vi "Test Asic Digital Offset modificar cluster.vi"(8 "Error IN":errorcluster, 11 "Config Test IN":T1={"Config HW"={"VISA Rigol DP832"="Rigol_DP832", "Config Rigol DP832"=[{"Channel"=0, "V Limit"=5.5, "I Limit"=0.5, "V Out"=5.0}, {"Channel"=1, "V Limit"=5.5, "I Limit"=0.8, "V Out"=5.0}, {"Channel"=2, "V Limit"=5.5, "I Limit"=0.2, "V Out"=0.0}], "CTA Test#"="CTA013 A", "FT_Handle"=0, "Espera acceso FT"=10}, "Config Test"=[{"Vasic"=3.3, "Test Register?"=TRUE, "Test ADC?"=TRUE, "Test ADC"={"Repeats ADC"=100, "Max Desviation"=0.1}, "Test Max PN Min NP?"=TRUE, "Limits Max PN Min NP"={"Max P inferior"=1.888, "Max P superior"=2.177000045776367, "Min N superior"=0.818, "Min N inferior"=0.73, "Max N superior"=1.475, "Max N inferior"=1.322, "Min P inferior "=1.321, "Min P superior"=1.474}, "Test Rate Scan?"=TRUE, "Vin Rate Scan"=[0, 1, 2, 3, 4, 5, 6, 7, 8, 9], "Limits Rate Scan"={"High"=[], "Low"=[]}, "Test Rate Scan Adders? 2"=FALSE, "Vin Rate Adders"=[], "Test offset analog?"=TRUE, "Test offset digital?"=FALSE, "Lim Offset Analog"={"Max Analog"=0.05, "Min Analog"=-0.05}, "Lim offset Dig"={"Max Dig"=0.05}}, {"Vasic"=3.2, "Test Register?"=TRUE, "Test ADC?"=TRUE, "Test ADC"={"Repeats ADC"=100, "Max Desviation"=0.1}, "Test Max PN Min NP?"=TRUE, "Limits Max PN Min NP"={"Max P inferior"=1.888, "Max P superior"=2.177000045776367, "Min N superior"=0.818, "Min N inferior"=0.73, "Max N superior"=1.475, "Max N inferior"=1.322, "Min P inferior "=1.321, "Min P superior"=1.474}, "Test Rate Scan?"=TRUE, "Vin Rate Scan"=[0, 3], "Limits Rate Scan"={"High"=[], "Low"=[]}, "Test Rate Scan Adders? 2"=FALSE, "Vin Rate Adders"=[], "Test offset analog?"=TRUE, "Test offset digital?"=FALSE, "Lim Offset Analog"={"Max Analog"=0.05, "Min Analog"=-0.05}, "Lim offset Dig"={"Max Dig"=0.05}}, {"Vasic"=3.1, "Test Register?"=TRUE, "Test ADC?"=TRUE, "Test ADC"={"Repeats ADC"=100, "Max Desviation"=0.1}, "Test Max PN Min NP?"=TRUE, "Limits Max PN Min NP"={"Max P inferior"=1.888, "Max P superior"=2.177000045776367, "Min N superior"=0.818, "Min N inferior"=0.73, "Max N superior"=1.475, "Max N inferior"=1.322, "Min P inferior "=1.321, "Min P superior"=1.474}, "Test Rate Scan?"=TRUE, "Vin Rate Scan"=[0, 3], "Limits Rate Scan"={"High"=[], "Low"=[]}, "Test Rate Scan Adders? 2"=FALSE, "Vin Rate Adders"=[], "Test offset analog?"=TRUE, "Test offset digital?"=FALSE, "Lim Offset Analog"={"Max Analog"=0.05, "Min Analog"=-0.05}, "Lim offset Dig"={"Max Dig"=0.05}}, {"Vasic"=3.0, "Test Register?"=TRUE, "Test ADC?"=TRUE, "Test ADC"={"Repeats ADC"=100, "Max Desviation"=0.1}, "Test Max PN Min NP?"=TRUE, "Limits Max PN Min NP"={"Max P inferior"=1.888, "Max P superior"=2.177000045776367, "Min N superior"=0.818, "Min N inferior"=0.73, "Max N superior"=1.475, "Max N inferior"=1.322, "Min P inferior "=1.321, "Min P superior"=1.474}, "Test Rate Scan?"=TRUE, "Vin Rate Scan"=[0, 3], "Limits Rate Scan"={"High"=[], "Low"=[]}, "Test Rate Scan Adders? 2"=FALSE, "Vin Rate Adders"=[], "Test offset analog?"=TRUE, "Test offset digital?"=FALSE, "Lim Offset Analog"={"Max Analog"=0.05, "Min Analog"=-0.05}, "Lim offset Dig"={"Max Dig"=0.05}}], "Result"=[], "Execucion Test"={"Vasic Actual"=0}, "Config VGA"={"Theoretical Voltage"=[], "Real Voltage"=[102.85, 207.14, 299.57, 404.85, 495.71, 606.85, 697.71, 801.14, 897.14, 998.85], "Pulse Width"=57344, "Frecuency Pulse"=1000000.0, "VGA Gain"=[9, 16, 24, 34, 43, 52, 61, 72, 81, 93]}, "Test Info"={"Asic"="", "Operator"="", "Time start"=timestamp(0 s since 1904-01-01), "Time stop"=timestamp(0 s since 1904-01-01)}} {"Config VGA"."Theoretical Voltage" format="%1.4f"; "Config VGA"."VGA Gain" format="%02x"; "Config VGA"."Frecuency Pulse" format="%0_2p"; "Config VGA"."Pulse Width" format="%04x"; "Config VGA"."Real Voltage" format="%1.5f"; "Config Test"."Lim offset Dig"."Max Dig" format="%.3g"; "Config Test"."Lim Offset Analog"."Min Analog" format="%.3g"; "Config Test"."Lim Offset Analog"."Max Analog" format="%.3g"; "Config Test"."Limits Rate Scan"."Low" format="%1.4f"; "Config Test"."Limits Rate Scan"."High" format="%1.3f"; "Config Test"."Limits Max PN Min NP"."Min P superior" format="%.3g"; "Config Test"."Limits Max PN Min NP"."Min P inferior" format="%.3g"; "Config Test"."Limits Max PN Min NP"."Max N inferior" format="%.3g"; "Config Test"."Limits Max PN Min NP"."Max N superior" format="%.3g"; "Config Test"."Limits Max PN Min NP"."Min N inferior" format="%.3g"; "Config Test"."Limits Max PN Min NP"."Min N superior" format="%.3g"; "Config Test"."Limits Max PN Min NP"."Max P superior" format="%.3g"; "Config Test"."Limits Max PN Min NP"."Max P inferior" format="%.3g"; "Config Test"."Vasic" min=2.8 max=3.8 step=0.01 format="%.2g"; "Config HW"."Config Rigol DP832"."Channel" items=["+30V Channel 1", "+30V Channel 2", "+5V Channel 3"]; "Config HW"."Config Rigol DP832"."V Limit" format="%.1g"; "Config HW"."Config Rigol DP832"."I Limit" format="%.1g"; "Config HW"."Config Rigol DP832"."V Out" format="%.1g"; "Result"."Test Registros"."Read W/R" format="%04x"; "Result"."Test Registros"."Pattern W/R" format="%04x"; "Result"."Test Registros"."Read Default" format="%04x"; "Result"."Test Registros"."Pattern Default" format="%04x"}) -> (0 "Error OUT":errorcluster, 3 "Config Test OUT":T1={"Config HW"={"VISA Rigol DP832"="Rigol_DP832", "Config Rigol DP832"=[{"Channel"=0, "V Limit"=5.5, "I Limit"=0.5, "V Out"=5.0}, {"Channel"=1, "V Limit"=5.5, "I Limit"=0.8, "V Out"=5.0}, {"Channel"=2, "V Limit"=5.5, "I Limit"=0.2, "V Out"=0.0}], "CTA Test#"="CTA013 A", "FT_Handle"=0, "Espera acceso FT"=10}, "Config Test"=[{"Vasic"=3.3, "Test Register?"=TRUE, "Test ADC?"=TRUE, "Test ADC"={"Repeats ADC"=100, "Max Desviation"=0.1}, "Test Max PN Min NP?"=TRUE, "Limits Max PN Min NP"={"Max P inferior"=1.888, "Max P superior"=2.177000045776367, "Min N superior"=0.818, "Min N inferior"=0.73, "Max N superior"=1.475, "Max N inferior"=1.322, "Min P inferior "=1.321, "Min P superior"=1.474}, "Test Rate Scan?"=TRUE, "Vin Rate Scan"=[0, 1, 2, 3, 4, 5, 6, 7, 8, 9], "Limits Rate Scan"={"High"=[], "Low"=[]}, "Test Rate Scan Adders? 2"=FALSE, "Vin Rate Adders"=[], "Test offset analog?"=TRUE, "Test offset digital?"=FALSE, "Lim Offset Analog"={"Max Analog"=0.05, "Min Analog"=-0.05}, "Lim offset Dig"={"Max Dig"=0.05}}, {"Vasic"=3.2, "Test Register?"=TRUE, "Test ADC?"=TRUE, "Test ADC"={"Repeats ADC"=100, "Max Desviation"=0.1}, "Test Max PN Min NP?"=TRUE, "Limits Max PN Min NP"={"Max P inferior"=1.888, "Max P superior"=2.177000045776367, "Min N superior"=0.818, "Min N inferior"=0.73, "Max N superior"=1.475, "Max N inferior"=1.322, "Min P inferior "=1.321, "Min P superior"=1.474}, "Test Rate Scan?"=TRUE, "Vin Rate Scan"=[0, 3], "Limits Rate Scan"={"High"=[], "Low"=[]}, "Test Rate Scan Adders? 2"=FALSE, "Vin Rate Adders"=[], "Test offset analog?"=TRUE, "Test offset digital?"=FALSE, "Lim Offset Analog"={"Max Analog"=0.05, "Min Analog"=-0.05}, "Lim offset Dig"={"Max Dig"=0.05}}, {"Vasic"=3.1, "Test Register?"=TRUE, "Test ADC?"=TRUE, "Test ADC"={"Repeats ADC"=100, "Max Desviation"=0.1}, "Test Max PN Min NP?"=TRUE, "Limits Max PN Min NP"={"Max P inferior"=1.888, "Max P superior"=2.177000045776367, "Min N superior"=0.818, "Min N inferior"=0.73, "Max N superior"=1.475, "Max N inferior"=1.322, "Min P inferior "=1.321, "Min P superior"=1.474}, "Test Rate Scan?"=TRUE, "Vin Rate Scan"=[0, 3], "Limits Rate Scan"={"High"=[], "Low"=[]}, "Test Rate Scan Adders? 2"=FALSE, "Vin Rate Adders"=[], "Test offset analog?"=TRUE, "Test offset digital?"=FALSE, "Lim Offset Analog"={"Max Analog"=0.05, "Min Analog"=-0.05}, "Lim offset Dig"={"Max Dig"=0.05}}, {"Vasic"=3.0, "Test Register?"=TRUE, "Test ADC?"=TRUE, "Test ADC"={"Repeats ADC"=100, "Max Desviation"=0.1}, "Test Max PN Min NP?"=TRUE, "Limits Max PN Min NP"={"Max P inferior"=1.888, "Max P superior"=2.177000045776367, "Min N superior"=0.818, "Min N inferior"=0.73, "Max N superior"=1.475, "Max N inferior"=1.322, "Min P inferior "=1.321, "Min P superior"=1.474}, "Test Rate Scan?"=TRUE, "Vin Rate Scan"=[0, 3], "Limits Rate Scan"={"High"=[], "Low"=[]}, "Test Rate Scan Adders? 2"=FALSE, "Vin Rate Adders"=[], "Test offset analog?"=TRUE, "Test offset digital?"=FALSE, "Lim Offset Analog"={"Max Analog"=0.05, "Min Analog"=-0.05}, "Lim offset Dig"={"Max Dig"=0.05}}], "Result"=[], "Execucion Test"={"Vasic Actual"=0}, "Config VGA"={"Theoretical Voltage"=[], "Real Voltage"=[102.85, 207.14, 299.57, 404.85, 495.71, 606.85, 697.71, 801.14, 897.14, 998.85], "Pulse Width"=57344, "Frecuency Pulse"=1000000.0, "VGA Gain"=[9, 16, 24, 34, 43, 52, 61, 72, 81, 93]}, "Test Info"={"Asic"="", "Operator"="", "Time start"=timestamp(0 s since 1904-01-01), "Time stop"=timestamp(0 s since 1904-01-01)}} {"Config VGA"."Theoretical Voltage" format="%1.4f"; "Config VGA"."VGA Gain" format="%02x"; "Config VGA"."Frecuency Pulse" format="%0_2p"; "Config VGA"."Pulse Width" format="%04x"; "Config VGA"."Real Voltage" format="%1.5f"; "Config Test"."Lim offset Dig"."Max Dig" format="%.3g"; "Config Test"."Lim Offset Analog"."Min Analog" format="%.3g"; "Config Test"."Lim Offset Analog"."Max Analog" format="%.3g"; "Config Test"."Limits Rate Scan"."Low" format="%1.4f"; "Config Test"."Limits Rate Scan"."High" format="%1.3f"; "Config Test"."Limits Max PN Min NP"."Min P superior" format="%.3g"; "Config Test"."Limits Max PN Min NP"."Min P inferior" format="%.3g"; "Config Test"."Limits Max PN Min NP"."Max N inferior" format="%.3g"; "Config Test"."Limits Max PN Min NP"."Max N superior" format="%.3g"; "Config Test"."Limits Max PN Min NP"."Min N inferior" format="%.3g"; "Config Test"."Limits Max PN Min NP"."Min N superior" format="%.3g"; "Config Test"."Limits Max PN Min NP"."Max P superior" format="%.3g"; "Config Test"."Limits Max PN Min NP"."Max P inferior" format="%.3g"; "Config Test"."Vasic" min=2.8 max=3.8 step=0.01 format="%.2g"; "Config HW"."Config Rigol DP832"."Channel" items=["+30V Channel 1", "+30V Channel 2", "+5V Channel 3"]; "Config HW"."Config Rigol DP832"."V Limit" format="%.1g"; "Config HW"."Config Rigol DP832"."I Limit" format="%.1g"; "Config HW"."Config Rigol DP832"."V Out" format="%.1g"; "Result"."Test Registros"."Read W/R" format="%04x"; "Result"."Test Registros"."Pattern W/R" format="%04x"; "Result"."Test Registros"."Read Default" format="%04x"; "Result"."Test Registros"."Pattern Default" format="%04x"})   [LabVIEW 2009]
uses:
  Test.ctl
  TEST.TEST CONFIG HW.ctl
  Rigol DP832/DP832_Control Channels.ctl
  TEST.TEST CONFIG TEST MATRIZ.ctl
  TEST.TEST CONFIG TEST.ctl
  TEST.TEST RESULT.ctl
  test_result fvasic.ctl
  TEST.TEST EXECUTION TEST.ctl
  TEST.TEST CONFIG VGA.ctl
  TEST.TEST TEST INFO.ctl
panel:
  out "REF":cluster{"Sumador":u8, "Canal":u8}
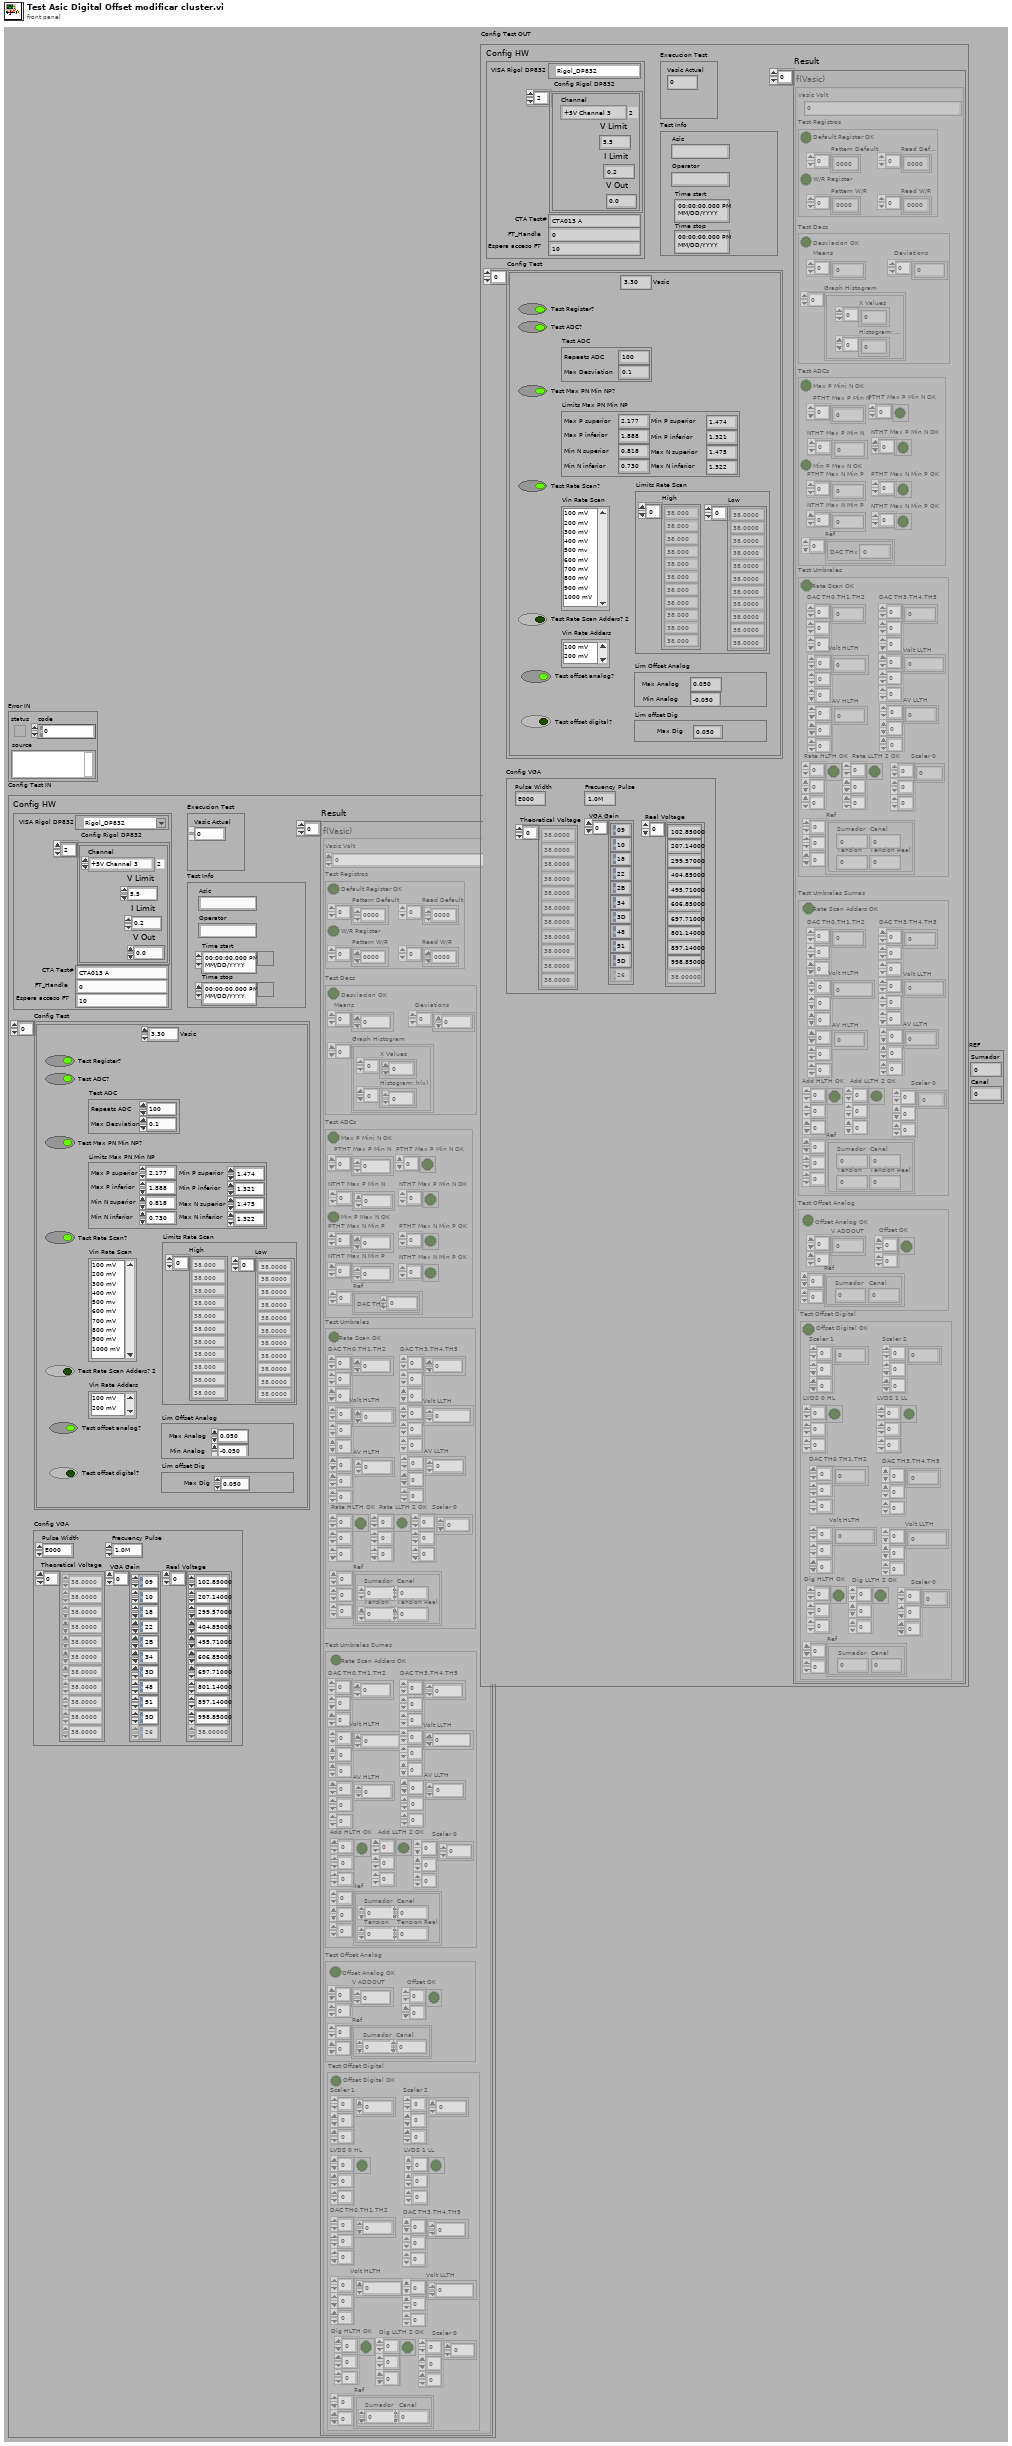
[diagram p1: front panel]
types:
  T1 = typedef "Test.ctl" = cluster{"Config HW":T2, "Config Test":T4, "Result":T6, "Execucion Test":T8, "Config VGA":T9, "Test Info":T10}
  T2 = typedef "TEST.TEST CONFIG HW.ctl" = cluster{"VISA Rigol DP832":refnum<visa-resource-name>, "Config Rigol DP832":cluster{"Channel":T3, "V Limit":dbl, "I Limit":dbl, "V Out":dbl}[], "CTA Test#":string, "FT_Handle":u32, "Espera acceso FT":u32}
  T3 = typedef "DP832_Control Channels.ctl" = i32
  T4 = typedef "TEST.TEST CONFIG TEST MATRIZ.ctl" = T5[]
  T5 = typedef "TEST.TEST CONFIG TEST.ctl" = cluster{"Vasic":dbl, "Test Register?":bool, "Test ADC?":bool, "Test ADC":cluster{"Repeats ADC":i32, "Max Desviation":dbl}, "Test Max PN Min NP?":bool, "Limits Max PN Min NP":cluster{"Max P inferior":dbl, "Max P superior":dbl, "Min N superior":dbl, "Min N inferior":dbl, "Max N superior":dbl, "Max N inferior":dbl, "Min P inferior ":dbl, "Min P superior":dbl}, "Test Rate Scan?":bool, "Vin Rate Scan":i32[], "Limits Rate Scan":cluster{"High":dbl[], "Low":dbl[]}, "Test Rate Scan Adders? 2":bool, "Vin Rate Adders":i32[], "Test offset analog?":bool, "Test offset digital?":bool, "Lim Offset Analog":cluster{"Max Analog":dbl, "Min Analog":dbl}, "Lim offset Dig":cluster{"Max Dig":dbl}}
  T6 = typedef "TEST.TEST RESULT.ctl" = T7[]
  T7 = typedef "test_result fvasic.ctl" = cluster{"Vasic Volt":i32, "Test Registros":cluster{"Default Register OK":bool, "Pattern Default":u16[], "Read Default":u16[], "W/R Register":bool, "Pattern W/R":u16[], "Read W/R":u16[]}, "Test Dacs":cluster{"Desviacion OK":bool, "Means":dbl[], "Deviations":dbl[], "Graph Histogram":cluster{"X Values":dbl[], "Histogram: h(x)":i32[]}[]}, "Test ADCs":cluster{"Max P Mini N OK":bool, "PTHT Max P Min N":dbl[], "PTHT Max P Min N OK":bool[], "NTHT Max P Min N":dbl[], "NTHT Max P Min N OK":bool[], "Min P Max N OK":bool, "PTHT Max N Min P":dbl[], "PTHT Max N Min P OK":bool[], "NTHT Max N Min P":dbl[], "NTHT Max N Min P OK":bool[], "Ref":cluster{"DAC THx":u8}[]}, "Test Umbrales":cluster{"Rate Scan OK":bool, "DAC TH0,TH1,TH2":u16[][][], "Volt HLTH":dbl[][][], "AV HLTH":dbl[][][], "Rate HLTH OK":bool[][][], "DAC TH3,TH4,TH5":u16[][][], "Volt LLTH":dbl[][][], "AV LLTH":dbl[][][], "Rate LLTH 2 OK":bool[][][], "Scaler 0":u16[][][], "Ref":cluster{"Sumador":u8, "Canal":u8, "Tension":u8, "Tension Real":dbl}[][][]}, "Test Umbrales Sumas":cluster{"Rate Scan Adders OK":bool, "DAC TH0,TH1,TH2":u16[][][], "Volt HLTH":dbl[][][], "AV HLTH":dbl[][][], "Add HLTH OK":bool[][][], "DAC TH3,TH4,TH5":u16[][][], "Volt LLTH":dbl[][][], "AV LLTH":dbl[][][], "Add LLTH 2 OK":bool[][][], "Scaler 0":u16[][][], "Ref":cluster{"Sumador":u8, "Canal":u8, "Tension":u8, "Tension Real":dbl}[][][]}, "Test Offset Analog":cluster{"Offset Analog OK":bool, "V ADDOUT":dbl[][], "Offset OK":bool[][], "Ref":cluster{"Sumador":u8, "Canal":u8}[][]}, "Test Offset Digital":cluster{"Offset Digital OK":bool, "Scaler 1":u16[][][], "LVDS 0 HL":bool[][][], "DAC TH0,TH1,TH2":u16[][][], "Volt HLTH":dbl[][][], "Dig HLTH OK":bool[][][], "Scaler 2":u16[][][], "LVDS 1 LL":bool[][][], "DAC TH3,TH4,TH5":u16[][][], "Volt LLTH":dbl[][][], "Dig LLTH 2 OK":bool[][][], "Scaler 0":u16[][][], "Ref":cluster{"Sumador":u8, "Canal":u8}[][]}}
  T8 = typedef "TEST.TEST EXECUTION TEST.ctl" = cluster{"Vasic Actual":i32}
  T9 = typedef "TEST.TEST CONFIG VGA.ctl" = cluster{"Theoretical Voltage":dbl[], "Real Voltage":dbl[], "Pulse Width":u16, "Frecuency Pulse":dbl, "VGA Gain":u8[]}
  T10 = typedef "TEST.TEST TEST INFO.ctl" = cluster{"Asic":string, "Operator":string, "Time start":timestamp, "Time stop":timestamp}
  T11 = cluster{"SCALER 0":u16[], "SCALER 1":u16[], "LVDS 1 HL":bool[], "THX":u16[], "VHLTH":dbl[], "SCALER 2":u16[], "LVDS 2 LL":bool[], "THX+3":u16[], "VLLTH":dbl[]}
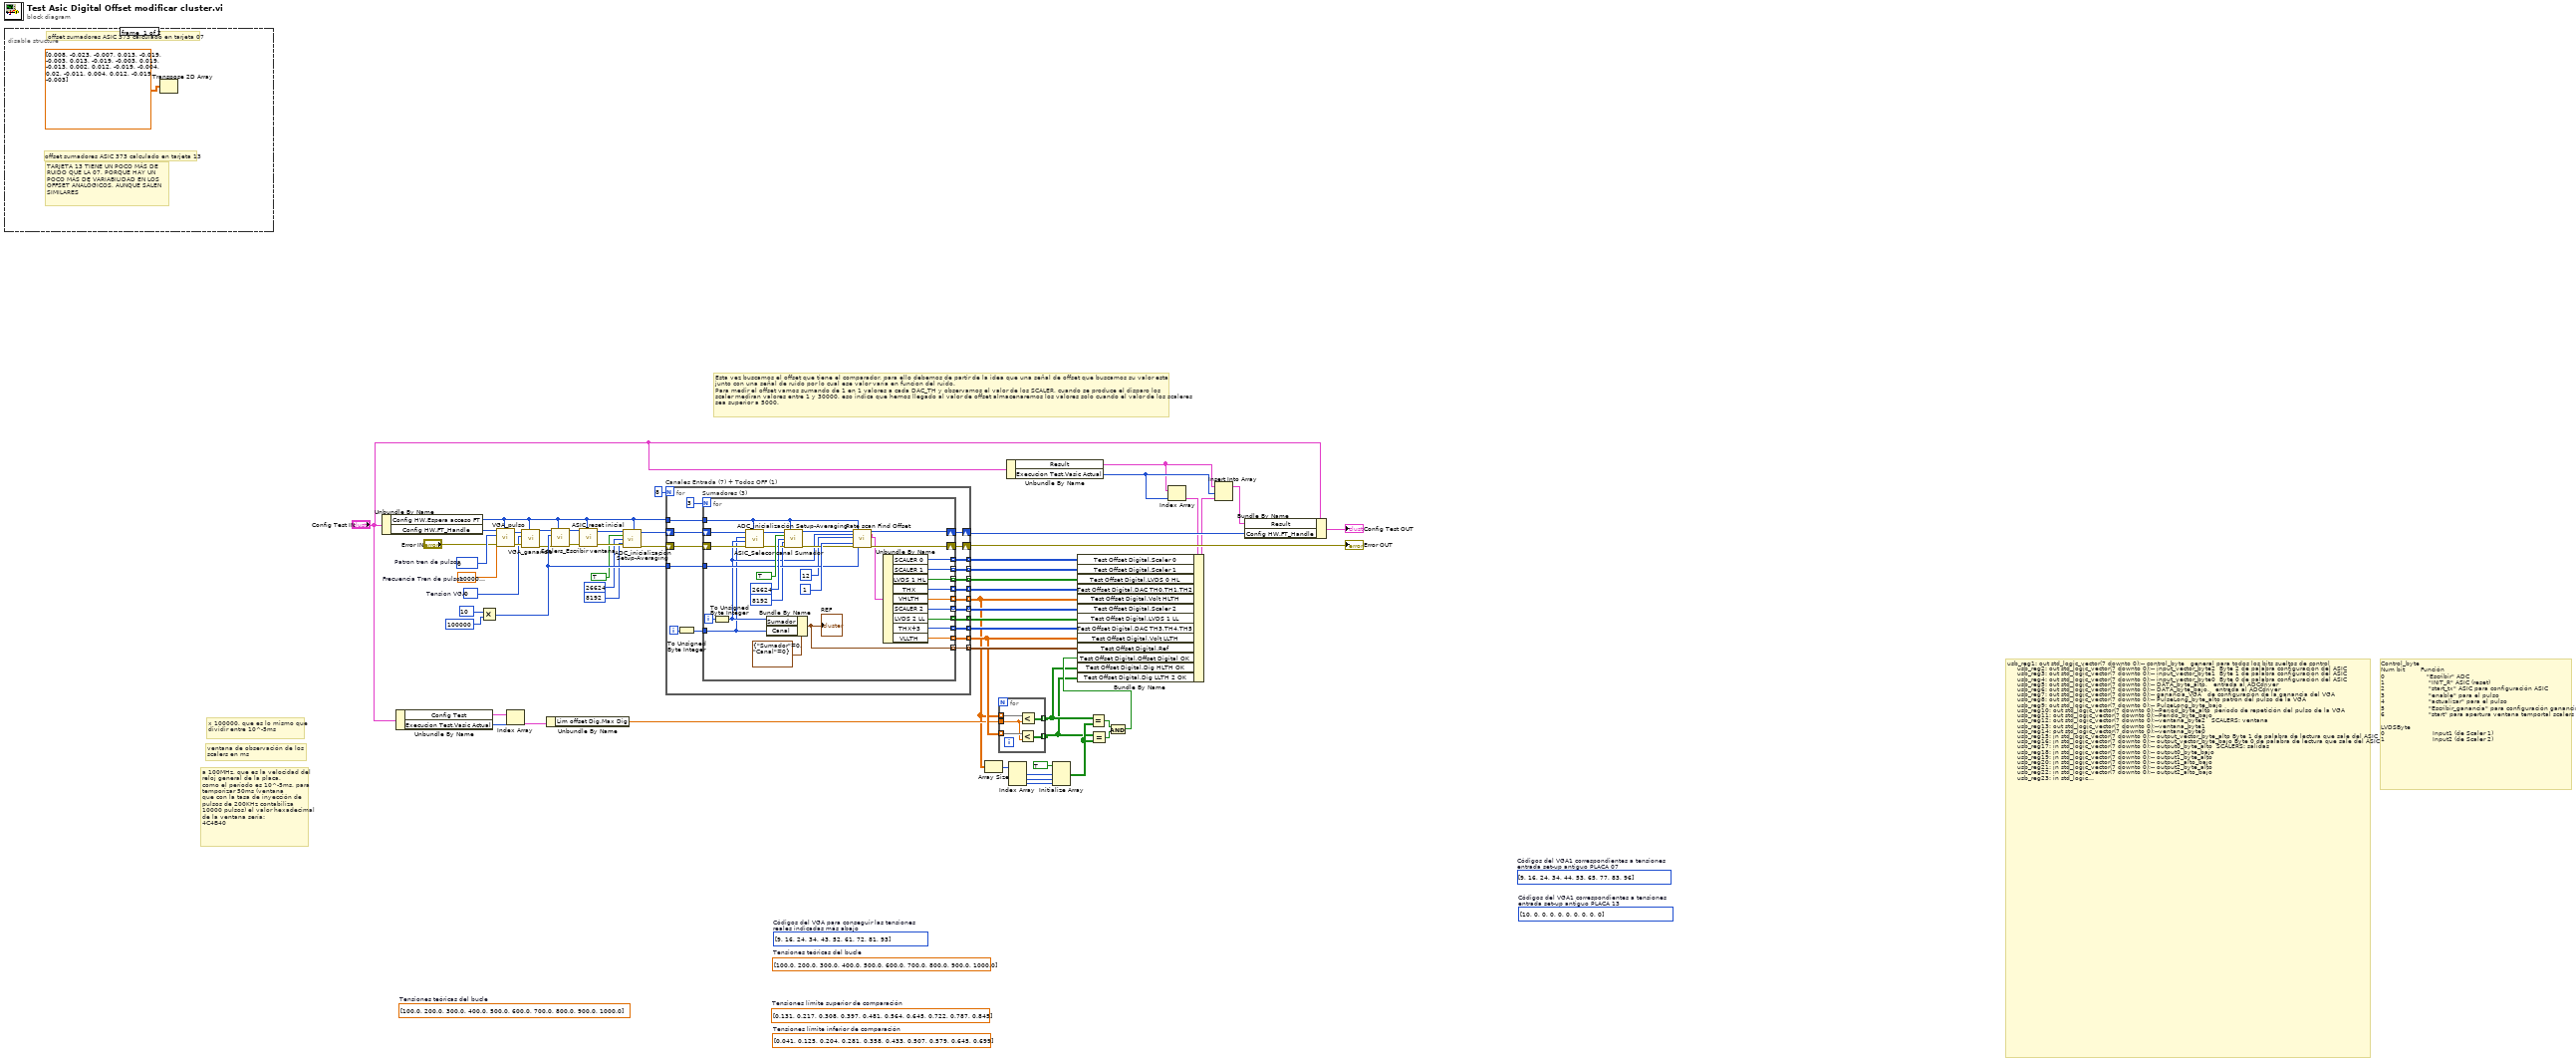
[diagram p0: block diagram]
diagram:
  w37 = u8 0  # Tension VGA
  (unwired) dbl[] [100.0, 200.0, 300.0, 400.0, 500.0, 600.0, 700.0, 800.0, 900.0, 1000.0]  # Tensiones teóricas del bucle
  w51 = 1000000.0  # Frecuencia Tren de pulsos
  w52 = u16 0  # Patron tren de pulsos
  (unwired) u8[] [10, 0, 0, 0, 0, 0, 0, 0, 0, 0]  # Códigos del VGA1 correspondientes a tensiones entrada set-up antiguo PLACA 13
  (unwired) u8[] [9, 16, 24, 34, 44, 53, 65, 77, 83, 96]  # Códigos del VGA1 correspondientes a tensiones entrada set-up antiguo PLACA 07
  (unwired) u8[] [9, 16, 24, 34, 43, 52, 61, 72, 81, 93]  # Códigos del VGA para conseguir las tensiones reales indicadas más abajo
  (unwired) dbl[] [0.041, 0.125, 0.204, 0.281, 0.358, 0.433, 0.507, 0.579, 0.645, 0.699]  # Tensiones límite inferior de comparación
  (unwired) dbl[] [0.131, 0.217, 0.308, 0.397, 0.481, 0.564, 0.645, 0.722, 0.787, 0.845]  # Tensiones límite superior de comparación
  (unwired) dbl[] [100.0, 200.0, 300.0, 400.0, 500.0, 600.0, 700.0, 800.0, 900.0, 1000.0]  # Tensiones teóricas del bucle
  # "Esta vez buscamos el offset que tiene el comparador, para ello debemos de partir de la idea que una señal de offset que buscamos su valor esta\njunto con una señal de ruido por lo cual ese valor varia en funcion del ruido.\nPara medir el offset vamos sumando de 1 en 1 valores a cada DAC_TH y observamos el valor de los SCALER, cuando se produce el disparo los\nscaler mediran valores entre 1 y 30000, eso indica que hemos llegado al valor de offset almacenaremos los valores solo cuando el valor de los scaleres\nsea superior a 5000."
  # "Control_byte\nNum bit        Función\n0                     \"Escribir\" ADC\n1                      \"INIT_R\" ASIC (reset)\n2                      \"start_tx\" ASIC para configuración ASIC\n3                      \"enable\" para el pulso\n4                      \"actualizar\" para el pulso\n5                      \"Escribir_ganancia\" para configuración ganancia\n6                      \"start\" para apertura ventana temportal scalers\n\nLVDSByte\n0                        Input1 (de Scaler 1)\n1                        Input2 (de Scaler 2)"
  # "usb_reg1: out std_logic_vector(7 downto 0);-- control_byte\t\t\tgeneral para todos los bits sueltos de control\n\t\t\t  usb_reg2: out std_logic_vector(7 downto 0);-- input_vector_byte2 \tByte 2 de palabra configuración del ASIC\n\t\t\t  usb_reg3: out std_logic_vector(7 downto 0);-- input_vector_byte1 \tByte 1 de palabra configuración del ASIC\n\t\t\t  usb_reg4: out std_logic_vector(7 downto 0);-- input_vector_byte0 \tByte 0 de palabra configuración del ASIC\n\t\t\t  usb_reg5: out std_logic_vector(7 downto 0);-- DATA_byte_alto, \t\tentrada al ADCdriver\n\t\t\t  usb_reg6: out std_logic_vector(7 downto 0);-- DATA_byte_bajo, \t\tentrada al ADCdriver\n\t\t\t  usb_reg7: out std_logic_vector(7 downto 0);-- ganancia_VGA\t\t\tde configuración de la ganancia del VGA\n\t\t\t  usb_reg8: out std_logic_vector(7 downto 0);-- PulseLong_byte_alto\tpatrón del pulso de la VGA\n\t\t\t  usb_reg9: out std_logic_vector(7 downto 0);-- PulseLong_byte_bajo\n\t\t\t  usb_reg10: out std_logic_vector(7 downto 0);--Period_byte_alto\t\tperíodo de repetición del pulso de la VGA\n\t\t\t  usb_reg11: out std_logic_vector(7 downto 0);--Perido_byte_bajo\n\t\t\t  usb_reg12: out std_logic_vector(7 downto 0);--ventana_byte2\t\t\tSCALERS: ventana\n\t\t\t  usb_reg13: out std_logic_vector(7 downto 0);--ventana_byte1\t\n\t\t\t  usb_reg14: out std_logic_vector(7 downto 0);--ventana_byte0\n\t\t\t  usb_reg15: in std_logic_vector(7 downto 0);-- output_vector_byte_alto\tByte 1 de palabra de lectura que sale del ASIC\n\t\t\t  usb_reg16: in std_logic_vector(7 downto 0);-- output_vector_byte_bajo\tByte 0 de palabra de lectura que sale del ASIC\n\t\t\t  usb_reg17: in std_logic_vector(7 downto 0);-- output0_byte_alto\t\tSCALERS: salidas\n\t\t\t  usb_reg18: in std_logic_vector(7 downto 0);-- output0_byte_bajo\n\t\t\t  usb_reg19: in std_logic_vector(7 downto 0);-- output1_byte_alto\n\t\t\t  usb_reg20: in std_logic_vector(7 downto 0);-- output1_alto_bajo \n\t\t\t  usb_reg21: in std_logic_vector(7 downto 0);-- output2_byte_alto \n\t\t\t  usb_reg22: in std_logic_vector(7 downto 0);-- output2_alto_bajo \n\t\t\t  usb_reg23: in std_logic_vector(7 downto 0);-- para el canal_0 del ADCdriver\n\t\t\t  usb_reg24: in std_logic_vector(7 downto 0);\n\t\t\t  usb_reg25: in std_logic_vector(7 downto 0);-- para el canal_1 del ADCdriver\n\t\t\t  usb_reg26: in std_logic_vector(7 downto 0);\n\t\t\t  usb_reg27: in std_logic_vector(7 downto 0);-- para el canal_2 del ADCdriver\n\t\t\t  usb_reg28: in std_logic_vector(7 downto 0);\n\t\t\t  usb_reg29: in std_logic_vector(7 downto 0);-- para el canal_3 del ADCdriver\n\t\t\t  usb_reg30: in std_logic_vector(7 downto 0);\n\t\t\t  usb_reg31: in std_logic_vector(7 downto 0);-- para el canal_4 del ADCdriver\n\t\t\t  usb_reg32: in std_logic_vector(7 downto 0);\n\t\t\t  usb_reg33: in std_logic_vector(7 downto 0);-- para el canal_5 del ADCdriver\n\t\t\t  usb_reg34: in std_logic_vector(7 downto 0);\n\t\t\t  usb_reg35: in std_logic_vector(7 downto 0);-- para el canal_6 del ADCdriver\n\t\t\t  usb_reg36: in std_logic_vector(7 downto 0);\n\t\t\t  usb_reg37: in std_logic_vector(7 downto 0);-- para el canal_7 del ADCdriver\n\t\t\t  usb_reg38: in std_logic_vector(7 downto 0);\n\t\t\t  usb_reg39: in std_logic_vector(7 downto 0);-- para el canal_8 del ADCdriver\n\t\t\t  usb_reg40: in std_logic_vector(7 downto 0);\n\t\t\t  usb_reg41: in std_logic_vector(7 downto 0);-- para el canal_9 del ADCdriver\n\t\t\t  usb_reg42: in std_logic_vector(7 downto 0);\n\t\t\t  usb_reg43: in std_logic_vector(7 downto 0);-- para el canal_10 del ADCdriver\n\t\t\t  usb_reg44: in std_logic_vector(7 downto 0)--;  \n\n     usb_reg55 => LVDSByte"
  # "x 100000, que es lo mismo que dividir entre 10^-5ms"
  # "ventana de observación de los scalers en ms"
  # "a 100MHz, que es la velocidad del reloj general de la placa,\ncomo el período es 10^-5ms, para temporizar 50ms (ventana \nque con la tasa de inyección de pulsos de 200KHz contabiliza \n10000 pulsos) el valor hexadecimal de la ventana sería:\n4C4B40"
  n1 = disable-structure shown="Enabled" {
    frame #0 {
      # "TARJETA 13 TIENE UN POCO MÁS DE \nRUIDO QUE LA 07, PORQUE HAY UN\nPOCO MÁS DE VARIABILIDAD EN LOS \nOFFSET ANALÓGICOS, AUNQUE SALEN\nSIMILARES"
      # "offset sumadores ASIC 373 calculado en tarjeta 13"
      # "offset sumadores ASIC 373 calculado en tarjeta 07"
      n2 = Transpose 2D Array(2D array=dbl[][] [[0.008, -0.023, -0.007], [0.013, -0.019, -0.003], [0.013, -0.019, -0.003], [0.019, -0.013, 0.002], [0.012, -0.019, -0.004], [0.02, -0.011, 0.004], [0.012, -0.019, -0.003]]) -> ()  [unwired: 1 out]
    }
    frame #1 {
    }
  }
  n3 = Unbundle By Name("Config Test IN") -> ("Config HW.Espera acceso FT"=w38:u32, "Config HW.FT_Handle"=w50:u32)
  n4 = Unbundle By Name("Config Test IN") -> ("Config Test"=w16:T4, "Execucion Test.Vasic Actual"=w17:i32)
  n5 = Multiply(x=u32 10 ("Ventana"), y=u32 100000 ("Ventana")) -> (x*y=w53:u32)
  n6 = call "VGA_pulso.vi"("Espera acceso USB"=w38, "error in"="Error IN", "Frecuencia pulso (0.2 a 1 Mhz)"=w51, "Patrón (E000)"=w52, "ftHandle_in"=w50) -> ("error out"=w42:errorcluster, "ftHandle_out"=w39:u32)  [unwired: 5 in]
  n7 = Index Array(array=w16, index=w17) -> (element=w15:T5)
  n8 = call "VGA_ganancia.vi"("Espera acceso USB"=w38, "error in 2"=w42, "Ganancia"=w37, "ftHandle_in 2"=w39) -> ("error out 2"=w41:errorcluster, "ftHandle_out 2"=w40:u32)  [unwired: 6 in]
  n9 = Unbundle By Name(w15) -> ("Lim offset Dig.Max Dig"=w13:dbl)
  n10 = call "Scalers_Escribir ventana.vi"("Espera acceso USB"=w38, "error in"=w41, "Ventana"=w53, "ftHandle_in"=w40) -> ("error out"=w54:errorcluster, "ftHandle_out"=w55:u32)  [unwired: 6 in]
  n11 = call "ASIC_reset inicial.vi"("Espera acceso USB"=w38, "error in"=w54, "ftHandle_in"=w55) -> ("error out"=w47:errorcluster, "ftHandle_out"=w48:u32)  [unwired: 7 in]
  n12 = call "ADC_inicialización Setup-Averaging.vi"("ftHandle_in 2"=w48, "Espera acceso USB"=w38, "Reset (T=reset)"=TRUE, "Registro Setup (0x6800)"=u16 26624, "Registro Averaging (0x3200)"=u16 8192 ("Registro Setup (0x6800)"), "error in 2"=w47) -> ("ftHandle_out"=w32:u32, "error out"=w31:errorcluster)  [unwired: 8 in]
  n13 = for "Canales Entrada (7) + Todos OFF (1)" {
    N: 8 -> [_]
    tunnel: w38 -> [w73]
    tunnel: w53 -> [w74]
    shift-right: [w70] -> w45
    shift-left: w32 -> [w77]
    shift-right: [w69] -> w46
    shift-left: w31 -> [w76]
    tunnel: [w68] -> w27 mode=indexing
    tunnel: [w67] -> w26 mode=indexing
    tunnel: [w66] -> w25 mode=indexing
    tunnel: [w65] -> w24 mode=indexing
    tunnel: [w64] -> w7 mode=indexing
    tunnel: [w63] -> w23 mode=indexing
    tunnel: [w62] -> w22 mode=indexing
    tunnel: [w61] -> w21 mode=indexing
    tunnel: [w60] -> w14 mode=indexing
    tunnel: [w59] -> w20 mode=indexing
    i -> [w75]
    n14 = To Unsigned Byte Integer(number=w75) -> (unsigned 8bit integer=w71:u8)
    n15 = for "Sumadores (3)" {
      N: 3 -> [_]
      tunnel: w71 -> [w79]
      tunnel: w74 -> [w101]
      tunnel: w73 -> [w96]
      shift-right: [w93] -> w69
      shift-left: w76 -> [w100]
      shift-right: [w94] -> w70
      shift-left: w77 -> [w99]
      tunnel: [w90] -> w68 mode=indexing
      tunnel: [w89] -> w67 mode=indexing
      tunnel: [w88] -> w66 mode=indexing
      tunnel: [w87] -> w65 mode=indexing
      tunnel: [w86] -> w64 mode=indexing
      tunnel: [w85] -> w63 mode=indexing
      tunnel: [w84] -> w62 mode=indexing
      tunnel: [w83] -> w61 mode=indexing
      tunnel: [w82] -> w60 mode=indexing
      tunnel: [w78] -> w59 mode=indexing
      i -> [w106]
      n16 = To Unsigned Byte Integer(number=w106) -> (unsigned 8bit integer=w80:u8)
      n17 = call "ASIC_Selecor canal Sumador.vi"("Espera acceso USB"=w96, "error in"=w100, "Sumador"=w80, "Canal"=w79, "ftHandle_in"=w99) -> ("error out"=w98:errorcluster, "ftHandle_out"=w97:u32)  [unwired: 4 in, 1 out]
      n18 = Bundle By Name(cluster=cluster{"Sumador":u8, "Canal":u8} {"Sumador"=0, "Canal"=0}, "Sumador"=w80, "Canal"=w79) -> (w78:cluster{"Sumador":u8, "Canal":u8})
      "REF" <- w78
      n19 = call "ADC_inicialización Setup-Averaging.vi"("ftHandle_in 2"=w97, "Espera acceso USB"=w96, "Reset (T=reset)"=TRUE, "Registro Setup (0x6800)"=u16 26624, "Registro Averaging (0x3200)"=u16 8192 ("Registro Setup (0x6800)"), "error in 2"=w98) -> ("ftHandle_out"=w103:u32, "error out"=w102:errorcluster)  [unwired: 8 in]
      n20 = call "Rate scan Find Offset.vi"("FtHander IN"=w103, "Sumador"=w80, "Max Recorido Dac"=12, "Valor buscado scalers (5000)"=u16 1 ("Valor buscado scalers"), "Error IN"=w102, "Espera acceso USB"=w96, "T Ventana"=w101) -> ("FtHander OUT"=w94:u32, "Todos los valores"=w91:T11, "Error OUT"=w93:errorcluster)  [unwired: 9 in, 1 out]
      n21 = Unbundle By Name(w91) -> ("SCALER 0"=w90:u16[], "SCALER 1"=w89:u16[], "LVDS 1 HL"=w88:bool[], "THX"=w87:u16[], "VHLTH"=w86:dbl[], "SCALER 2"=w85:u16[], "LVDS 2 LL"=w84:bool[], "THX+3"=w83:u16[], "VLLTH"=w82:dbl[])
    }
  }
  "Error OUT" <- w46
  n22 = Array Size(array=w7) -> (size(s)=w12:i32[])
  n23 = for {
    tunnel: w7 -> [w112] mode=indexing
    tunnel: w14 -> [w111] mode=indexing
    tunnel: w13 -> [w110]
    tunnel: [w109] -> w2 mode=indexing
    tunnel: [w108] -> w1 mode=indexing
    n24 = Less?(x=w111, y=w110) -> (x < y?=w108:bool[][])
    n25 = Less?(x=w112, y=w110) -> (x < y?=w109:bool[][])
  }
  n26 = Unbundle By Name("Config Test IN") -> ("Result"=w30:T6, "Execucion Test.Vasic Actual"=w43:i32)
  n27 = Index Array(array=w12) -> (element #1=w11:i32, element #2=w10:i32, element #3=w9:i32)  [unwired: 3 in]
  n28 = Initialize Array(TRUE, w11, w10, w9) -> (w4:bool[][][])
  n29 = Equal?(x=w2, y=w4) -> (x = y?=w6:bool)
  n30 = Equal?(x=w1, y=w4) -> (x = y?=w5:bool)
  n31 = And(x=w6, y=w5) -> (x .and. y?=w3:bool)
  n32 = Index Array(array=w30, index=w43) -> (element=w28:T7)
  n33 = Bundle By Name(cluster=w28, "Test Offset Digital.Scaler 0"=w27, "Test Offset Digital.Scaler 1"=w26, "Test Offset Digital.LVDS 0 HL"=w25, "Test Offset Digital.DAC TH0,TH1,TH2"=w24, "Test Offset Digital.Volt HLTH"=w7, "Test Offset Digital.Scaler 2"=w23, "Test Offset Digital.LVDS 1 LL"=w22, "Test Offset Digital.DAC TH3,TH4,TH5"=w21, "Test Offset Digital.Volt LLTH"=w14, "Test Offset Digital.Ref"=w20, "Test Offset Digital.Offset Digital OK"=w3, "Test Offset Digital.Dig HLTH OK"=w2, "Test Offset Digital.Dig LLTH 2 OK"=w1) -> (w19:T7)
  n34 = Insert Into Array(array=w30, index=w43, new element=w19) -> (w29:T6)
  n35 = Bundle By Name(cluster="Config Test IN", "Result"=w29, "Config HW.FT_Handle"=w45) -> (→"Config Test OUT":T1)
